vi "writeVESC.vi"(1 "ID":u32 format="%x", 2 "Control Value":fxp<+/-,32,16>, 3 "Control Mode":T2(ring), 4 "SPI Config In":T1) -> (0 "SPI Config Out":T1)   [LabVIEW 2019]
uses:
  SPI/SPI Config.ctl
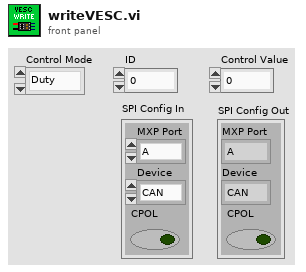
[diagram p1: front panel]
types:
  T1 = typedef "SPI Config.ctl" = cluster{"MXP Port":enum16{"A", "B"}, "Device":enum16{"CAN", "ENC", "IMU1", "IMU2"}, "CPOL":bool}
  T2 = enum32{"Duty", "Current", "Brake", "RPM", "Position"}
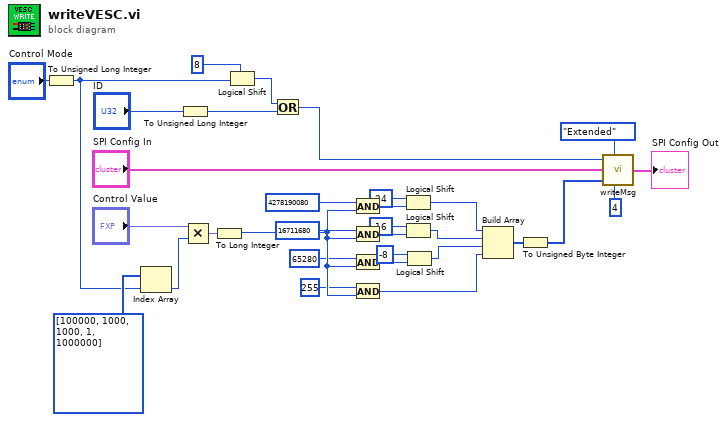
[diagram p0: block diagram]
diagram:
  n1 = To Unsigned Long Integer(number="Control Mode") -> (unsigned 32bit integer=w7:u32)
  n2 = Index Array(array=i32[] [100000, 1000, 1000, 1, 1000000], index=w7) -> (element=w9:i32)
  n3 = To Unsigned Long Integer(number="ID") -> (unsigned 32bit integer=w29:u32)
  n4 = Multiply(x="Control Value", y=w9) -> (x*y=w27:fxp<+/-,64,48>)
  n5 = To Long Integer(number=w27) -> (32bit integer=w26:i32)
  n6 = Logical Shift(y=i16 8, x=w7) -> (x << y=w31:u32)
  n7 = Or(x=w31, y=w29) -> (x .or. y?=w5:u32)
  n8 = And(x=u32 4278190080, y=w26) -> (x .and. y?=w21:u32)
  n9 = And(x=u32 16711680, y=w26) -> (x .and. y?=w20:u32)
  n10 = And(x=u32 65280, y=w26) -> (x .and. y?=w19:u32)
  n11 = And(x=u32 255, y=w26) -> (x .and. y?=w12:u32)
  n12 = Logical Shift(y=i16 -24, x=w21) -> (x << y=w15:u32)
  n13 = Logical Shift(y=i16 -16, x=w20) -> (x << y=w14:u32)
  n14 = Logical Shift(y=i16 -8, x=w19) -> (x << y=w13:u32)
  n15 = Build Array(w15, w14, w13, w12) -> (w11:u32[])
  n16 = To Unsigned Byte Integer(number=w11) -> (unsigned 8bit integer=w4:u8[])
  n17 = call "writeMsg.vi"("ID"=w5, "ID Type"=enum16{"Standard", "Extended"}."Extended", "SPI Config In"="SPI Config In", "Data to Write"=w4, "Frames to Write"=u8 4) -> ("SPI Config Out"=→"SPI Config Out":T1)
